vi "задача 2.vi"() -> ()   [LabVIEW 2019]
uses:
  <vilib>/myRIO/Express VI/Onboard IO/DI/DI Express VI.xnode
  <vilib>/myRIO/Instrument Drivers/Onboard IO/DIO/vis/Read.vi
  <vilib>/myRIO/Instrument Drivers/Onboard IO/DIO/DIO.lvlib
  <vilib>/myRIO/Common/Instrument Driver Framework/myRIO v1.0/DIO/typedefs/DIO Channels Enum.ctl
  <vilib>/myRIO/Common/Instrument Driver Framework/myRIO v1.0/DIO/typedefs/DIO Channels List.ctl
  <vilib>/myRIO/Common/Instrument Driver Framework/Utilities/typedefs/Generic FPGA Reference.ctl
  <vilib>/myRIO/Common/Instrument Driver Framework/Utilities/typedefs/myRIO v1.0 Reference.ctl
  <vilib>/myRIO/Common/Instrument Driver Framework/Utilities/typedefs/Hardware Version Enum.ctl
  <vilib>/myRIO/Common/Instrument Driver Framework/Utilities/typedefs/myRIO Generic Hardware Reference.ctl
  <vilib>/myRIO/Instrument Drivers/Onboard IO/DIO/typedefs/DIO Reference.ctl
  <vilib>/myRIO/Instrument Drivers/Onboard IO/DIO/vis/myRIO DIO Open.xnode
  <vilib>/myRIO/Common/Instrument Driver Framework/Utilities/vis/Is FPGA Ref Available.vi
  <vilib>/myRIO/Common/Instrument Driver Framework/myRIO v1.0/DIO/vis/myRIO v1.1 Open DIO.vi
  <vilib>/userDefined/High Color/nirio_resource_hc.ctl
  <vilib>/myRIO/Express VI/Onboard Devices/LED/LED Express VI.xnode
  <vilib>/myRIO/Instrument Drivers/Onboard IO/DIO/vis/Write.vi
  <vilib>/myRIO/Express VI/Onboard IO/DO/DO Express VI.xnode
panel:
  out "Numeric 2":dbl
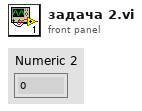
[diagram p1: front panel]
types:
  T1 = typedef "DIO.lvlib/DIO Reference.ctl" = cluster{"myRIO Reference":T2, "DIO Channels List":T6}
  T2 = typedef "myRIO Generic Hardware Reference.ctl" = cluster{"myRIO Model":T3, "myRIO Hardware Reference":T4}
  T3 = typedef "Hardware Version Enum.ctl" = enum16{"Unknown", "myRIO-1900", "myRIO-1950", "roboRIO", "NI ELVIS RIO CM", "ELVIS III"}
  T4 = typedef "myRIO v1.0 Reference.ctl" = cluster{"Generic FPGA Reference":T5, "Allow multiple opens":bool}
  T5 = typedef "Generic FPGA Reference.ctl" = refnum<k20>
  T6 = typedef "DIO Channels List.ctl" = T7[]
  T7 = typedef "DIO Channels Enum.ctl" = enum16{"Not Connected", "C/DIO0", "C/DIO1", "C/DIO2", "C/DIO3", "C/DIO4", "C/DIO5", "C/DIO6", "C/DIO7", "A/DIO0", "A/DIO1", "A/DIO2", "A/DIO3", "A/DIO4", "A/DIO5", "A/DIO6", "A/DIO7", "A/DIO8", "A/DIO9", "A/DIO10", "A/DIO11", "A/DIO12", "A/DIO13", "A/DIO14", "A/DIO15", "A/DIO16", "A/DIO17", "A/DIO18", "A/DIO19", "B/DIO0", "B/DIO1", "B/DIO2", "B/DIO3", "B/DIO4", "B/DIO5", "B/DIO6", "B/DIO7", "B/DIO8", "B/DIO9", "B/DIO10", "B/DIO11", "B/DIO12", "B/DIO13", "B/DIO14", "B/DIO15", "B/DIO16", "B/DIO17", "B/DIO18", "B/DIO19", "LED0", "LED1", "LED2", "LED3", "Button0", "DIO/DIO0", "DIO/DIO1", "DIO/DIO2", "DIO/DIO3", "DIO/DIO4", "DIO/DIO5", "DIO/DIO6", "DIO/DIO7", "DIO/DIO8", "DIO/DIO9", "SPI/CS0", "SPI/CS1", "SPI/CS2", "SPI/CS3", "LED RADIO (Green)", "LED RADIO (Red)", "LED COMM (Green)", "LED COMM (Red)", "LED MODE (Green)", "LED MODE (Red)"}
  T8 = typedef "nirio_resource_hc.ctl" = tag
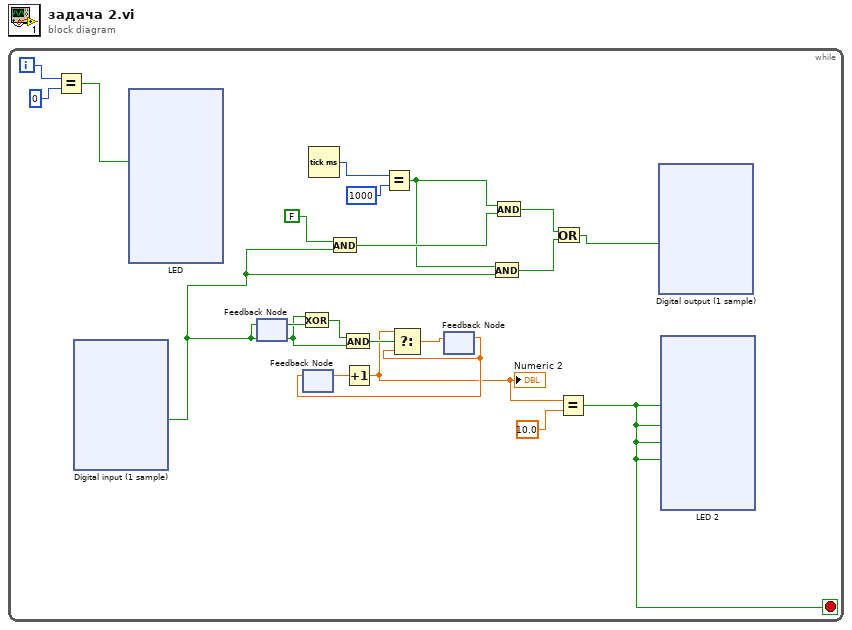
[diagram p0: block diagram]
diagram:
  n1 = while {
    i -> [w19]
    stop <- w1 stop-if-true
    n2 = Equal?(x=w19, y=0 ("x")) -> (x = y?=w17:bool)
    n3 = xnode "Digital input (1 sample)"() -> ("A/DIO0 (Pin 11)"=w4:bool)  [unwired: 1 in, 1 out]
    n4 = xnode "LED"("LED0"=w17) -> ()  [unwired: 4 in, 1 out]
    n5 = feedback #1() -> (w7:bool)  [unwired: 1 in]
    n6 = feedback-in #1(w4) -> ()
    n7 = Exclusive Or(1:w7, 2:w4) -> (0:w6:bool)
    n8 = feedback #2() -> (w10:dbl)  [unwired: 1 in]
    n9 = Tick Count (ms)() -> (millisecond timer value=w21:u32)
    n10 = And(x=FALSE, y=w4) -> (x .and. y?=w15:bool)
    n11 = And(x=w6, y=w4) -> (x .and. y?=w5:bool)
    n12 = Increment(x=w10) -> (x+1=w3:dbl)
    "Numeric 2" <- w3
    n13 = Equal?(x=w21, y=u32 1000 ("x")) -> (x = y?=w14:bool)
    n14 = feedback #3() -> (w8:dbl)  [unwired: 1 in]
    n15 = feedback-in #2(w8) -> ()
    n16 = Select(t=w3, s=w5, f=w8) -> (s? t:f=w9:dbl)
    n17 = feedback-in #3(w9) -> ()
    n18 = And(x=w14, y=w4) -> (x .and. y?=w13:bool)
    n19 = And(x=w14, y=w15) -> (x .and. y?=w12:bool)
    n20 = Or(x=w12, y=w13) -> (x .or. y?=w11:bool)
    n21 = Equal?(x=w3, y=10.0 ("x")) -> (x = y?=w1:bool)
    n22 = xnode "Digital output (1 sample)"("A/DIO1 (Pin 13)"=w11) -> ()  [unwired: 1 in, 1 out]
    n23 = xnode "LED 2"("LED0"=w1, "LED1"=w1, "LED2"=w1, "LED3"=w1) -> ()  [unwired: 1 in, 1 out]
  }
